vi "picoscopeInitializeSettings.vi"(6 "nSegmentsInt":i32, 7 "nSegments":T2 format="%.4p", 8 "error in (no error)":errorcluster, 9 "Use Serial Number":bool, 10 "Serial Number":string, 11 "PicoscopeV2 in":refnum<class "PicoscopeV2.lvclass">) -> (0 "error out":errorcluster, 1 "Device Info":T1, 2 "USB 3.0 device on non-USB 3.0 Port":bool, 3 "PicoscopeV2 out":refnum<class "PicoscopeV2.lvclass">, 5 "USB Powered":bool=TRUE)   [LabVIEW 2020, in "PicoscopeV2.lvclass"]
uses:
  PicoscopeV2.lvclass
  nSegments.ctl
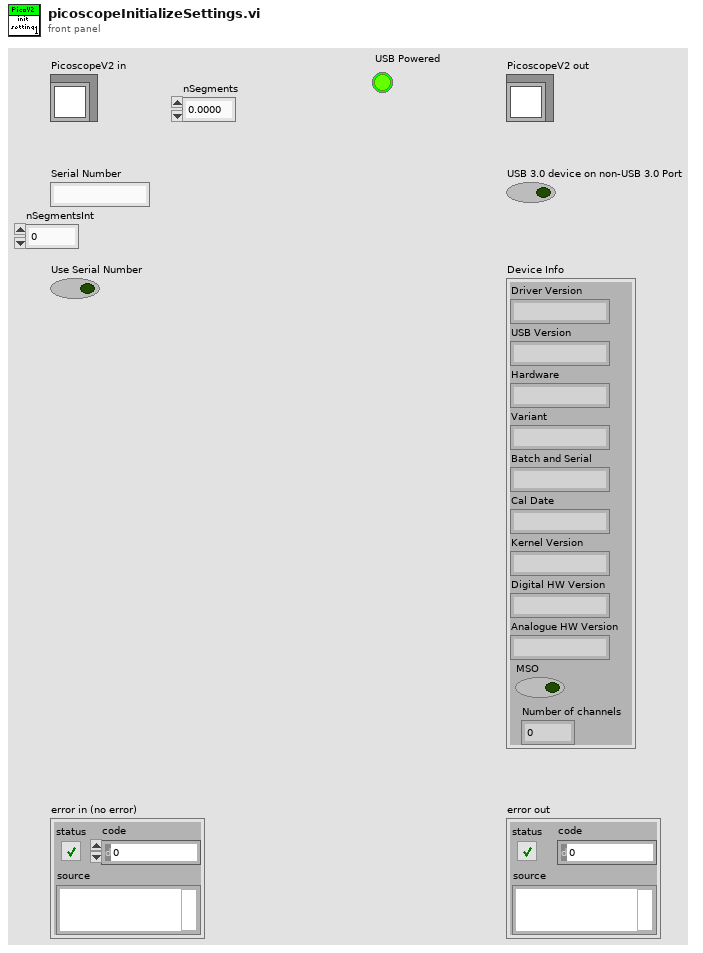
[diagram p1: front panel]
types:
  T1 = cluster{"Driver Version":string, "USB Version":string, "Hardware":string, "Variant":string, "Batch and Serial":string, "Cal Date":string, "Kernel Version":string, "Digital HW Version":string, "Analogue HW Version":string, "MSO":bool, "Number of channels":i16}
  T2 = typedef "nSegments.ctl" = u64
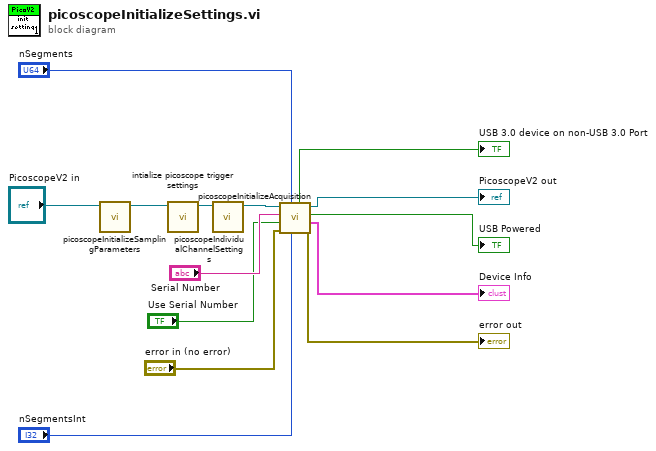
[diagram p0: block diagram]
diagram:
  n1 = call-dynamic "picoscopeInitializeSamplingParameters.vi"("PicoscopeV2 in"="PicoscopeV2 in") -> ("PicoscopeV2 out"=w3:refnum<class "PicoscopeV2.lvclass">)  [unwired: 10 in]
  n2 = call-dynamic "intialize picoscope trigger settings.vi"("PicoscopeV2 in"=w3) -> ("PicoscopeV2 out"=w6:refnum<class "PicoscopeV2.lvclass">)  [unwired: 10 in]
  n3 = call-dynamic "picoscopeIndividualChannelSettings.vi"("PicoscopeV2 in"=w6) -> ("PicoscopeV2 out"=w5:refnum<class "PicoscopeV2.lvclass">)  [unwired: 10 in]
  n4 = call-dynamic "picoscopeInitializeAcquisition.vi"("nSegmentsInt"="nSegmentsInt", "nSegments"="nSegments", "error in (no error)"="error in (no error)", "Use Serial Number"="Use Serial Number", "Serial Number"="Serial Number", "PicoscopeV2 in"=w5) -> ("error out"=→"error out":errorcluster, "Device Info"=→"Device Info":T1, "USB Powered"=→"USB Powered":bool, "PicoscopeV2 out"=→"PicoscopeV2 out":refnum<class "PicoscopeV2.lvclass">, "USB 3.0 device on non-USB 3.0 Port"=→"USB 3.0 device on non-USB 3.0 Port":bool)  [unwired: 1 out]
